vi "VISA MEMACC Read U8 vs U64.vi"() -> ()   [LabVIEW 2016]
uses:
  <vilib>/Platform/TimedLoop/XDataNode/timing_clust.ctl
  <vilib>/Platform/TimedLoop/XDataNode/nitl_modes.ctl
  <vilib>/Platform/TimedLoop/XDataNode/wakeup.ctl
  Source/GE 5565PIORC/GE 5565PIORC Old.lvclass/GE 5565PIORC Old.ctl
  Source/GE 5565PIORC/VIs/Block Operations/Allocate Single Block.vi
  Source/GE 5565PIORC/VIs/Registers/Local Configuration.LAS1RR.Address Range.Get.vi
  Source/GE 5565PIORC/VIs/Binary Operations/Align to 8-byte Boundary.vi
  Source/GE 5565PIORC/VIs/Binary Operations/Align to 16-byte Boundary.vi
  Source/GE 5565PIORC/VIs/Registers/Local Configuration.Get Register Offset.vi
  Source/GE 5565PIORC/GE 5565PIORC Old.lvclass
  <vilib>/platform/TimedLoop/XDataNode/XDataNode.xnode
  <vilib>/Platform/TimedLoop/XDataNode/XDNodeRunTimeDep.lvlib
panel:
  out "U64 Duration":dbl
  in  "U64s":i32
  out "U8 Duration":dbl
  in  "VISA resource name":refnum<visa-resource-name>
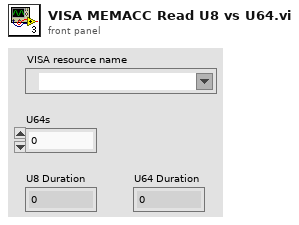
[diagram p1: front panel]
types:
  T1 = typedef "XDNodeRunTimeDep.lvlib/timing_clust.ctl" = cluster{"Expected End [f-1]":u64, "Actual End [f-1]":u64, "Finished Late? [f-1]":bool, "Expected End [i-1]":u64, "Actual End [i-1]":u64, "Finished Late? [i-1]":bool, "Expected Start [i]":u64, "Actual Start [i]":u64, "Expected Start [f]":u64, "Actual Start [f]":u64, "Source Name":string, "Structure Name":string, "Period":i64, "Deadline":i64, "Offset":i64, "Start":i64, "Priority":i32, "Timeout":i32, "Mode":T2, "Wakeup Reason":T3, "Error":errorcluster, "Source Type":string, "Secondary Source Type":string, "Global End Time":u64, "Global Start Time":u64, "Frame Duration":u64, "Iteration Duration":u64, "Assigned CPU":i32, "I/O Scan Engine Mode":u32}
  T2 = typedef "XDNodeRunTimeDep.lvlib/nitl_modes.ctl" = enum32{"No Change", "Process missed periods, maintain original phase", "Discard missed periods, maintain original phase", "Process missed periods, ignore original phase", "Discard missed periods, ignore original phase"}
  T3 = typedef "XDNodeRunTimeDep.lvlib/wakeup.ctl" = enum32{"Normal", "Aborted", "Asynchronous wakeup", "Timing source error", "Timed loop error", "Timeout"}
  T4 = typedef "GE 5565PIORC Old.lvclass/DMA Block Descriptor.ctl" = cluster{"descriptor ptr (VISA)":u32, "descriptor size":u32, "descriptor ptr (aligned)":u32, "data ptr (lower)":u32, "data ptr (upper)":u32, "data size":u32, "next descriptor ptr":u32}
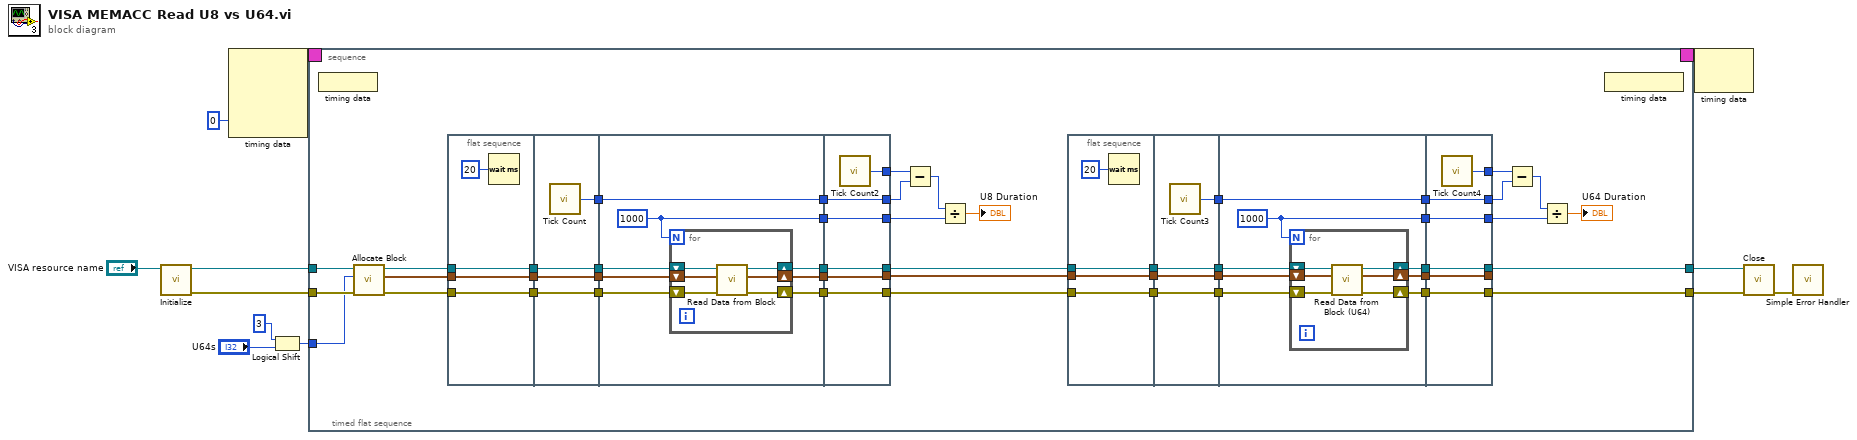
[diagram p0: block diagram]
diagram:
  n1 = call "Initialize.vi"("VISA resource name"="VISA resource name") -> ("error out"=w6:errorcluster, "GE 5565PIORC"=w7:refnum<class "GE 5565PIORC Old.lvclass">)  [unwired: 9 in]
  n2 = node-c288(0 ("Processor")) -> (w10:T1)  [unwired: 3 in]
  n3 = Logical Shift(y=i16 3, x="U64s") -> (x << y=w4:i32)
  n4 = timed-sequence {
    timing: w10 -> [_]
    timing-out: [_] -> w9
    tunnel: w7 -> [w14]
    tunnel: w6 -> [w17]
    tunnel: [w16] -> w1
    tunnel: w4 -> [w15]
    tunnel: [w13] -> w2
    n5 = timed-flat-sequence {
      tunnel: w17 -> [w35]
      tunnel: [w37] -> w16
      tunnel: w15 -> [w32]
      tunnel: w14 -> [w36]
      tunnel: [w18] -> w13
      n6 = node-c288() -> ()  [unwired: 1 in]
      n7 = call-poly "Allocate Block.vi"("error in (no error)"=w35, "size (bytes)"=w32, "GE 5565PIORC in"=w36) -> ("error out"=w33:errorcluster, "Block Descriptor"=w27:T4, "GE 5565PIORC out"=w34:refnum<class "GE 5565PIORC Old.lvclass">)  [unwired: 6 in]
      n8 = flat-sequence {
        tunnel: w34 -> [w93]
        tunnel: w33 -> [w92]
        tunnel: [w93] -> w57
        tunnel: [w92] -> w55
        tunnel: w27 -> [w91]
        tunnel: [w91] -> w26
        tunnel: [w98] -> w62
        tunnel: [w97] -> w58
        tunnel: w57 -> [w97]
        tunnel: [w96] -> w56
        tunnel: w55 -> [w96]
        tunnel: w26 -> [w95]
        tunnel: [w95] -> w25
        tunnel: w62 -> [w106]
        tunnel: [w106] -> w61
        tunnel: w58 -> [w103]
        tunnel: w56 -> [w102]
        tunnel: [w105] -> w54
        tunnel: [w104] -> w53
        tunnel: [w101] -> w31
        tunnel: w25 -> [w100]
        tunnel: [w99] -> w24
        tunnel: [w118] -> w60
        tunnel: [w117] -> w59
        tunnel: w61 -> [w117]
        tunnel: w54 -> [w116]
        tunnel: [w116] -> w38
        tunnel: w53 -> [w115]
        tunnel: [w115] -> w51
        tunnel: w31 -> [w114]
        tunnel: [w114] -> w28
        tunnel: w24 -> [w113]
        tunnel: [w113] -> w23
        frame #0 {
          n9 = Wait (ms)(milliseconds to wait=u32 20) -> ()  [unwired: 1 out]
        }
        frame #1 {
          n10 = call "Tick Count"() -> ("Tick Count(uSec)"=w98:u32)
        }
        frame #2 {
          w104 = 1000
          n11 = for {
            N: w104 -> [_]
            shift-right: [w111] -> w101
            shift-left: w103 -> [w112]
            shift-right: [w109] -> w105
            shift-left: w102 -> [w110]
            shift-right: [w107] -> w99
            shift-left: w100 -> [w108]
            n12 = call "Read Data from Block.vi"("error in (no error)"=w110, "Block Descriptor"=w108, "GE 5565PIORC"=w112) -> ("error out"=w109:errorcluster, "Block Descriptor out"=w107:T4, "GE 5565PIORC out"=w111:refnum<class "GE 5565PIORC Old.lvclass">)  [unwired: 5 in, 1 out]
          }
        }
        frame #3 {
          n13 = call "Tick Count2"() -> ("Tick Count(uSec)"=w118:u32)
        }
      }
      n14 = Subtract(x=w60, y=w59) -> (x-y=w52:u32)
      n15 = Divide(x=w52, y=w51) -> (x/y=→"U8 Duration":dbl)
      n16 = flat-sequence {
        tunnel: w38 -> [w65]
        tunnel: [w65] -> w49
        tunnel: [w64] -> w29
        tunnel: w28 -> [w64]
        tunnel: w23 -> [w63]
        tunnel: [w63] -> w22
        tunnel: [w70] -> w48
        tunnel: [w69] -> w47
        tunnel: w49 -> [w69]
        tunnel: [w68] -> w30
        tunnel: w29 -> [w68]
        tunnel: w22 -> [w67]
        tunnel: [w67] -> w21
        tunnel: w48 -> [w78]
        tunnel: [w78] -> w46
        tunnel: w47 -> [w73]
        tunnel: [w77] -> w45
        tunnel: [w76] -> w44
        tunnel: w30 -> [w75]
        tunnel: w21 -> [w74]
        tunnel: [w72] -> w20
        tunnel: [w71] -> w19
        tunnel: [w90] -> w43
        tunnel: [w89] -> w42
        tunnel: w46 -> [w89]
        tunnel: w45 -> [w88]
        tunnel: [w88] -> w37
        tunnel: w44 -> [w87]
        tunnel: [w87] -> w40
        tunnel: w20 -> [w85]
        tunnel: w19 -> [w86]
        tunnel: [w86] -> w18
        tunnel: [w85] -> _
        frame #0 {
          n17 = Wait (ms)(milliseconds to wait=u32 20) -> ()  [unwired: 1 out]
        }
        frame #1 {
          n18 = call "Tick Count3"() -> ("Tick Count(uSec)"=w70:u32)
        }
        frame #2 {
          w76 = 1000
          n19 = for {
            N: w76 -> [_]
            shift-right: [w81] -> w77
            shift-left: w73 -> [w82]
            shift-right: [w80] -> w71
            shift-left: w75 -> [w84]
            shift-right: [w79] -> w72
            shift-left: w74 -> [w83]
            n20 = call "Read Data from Block (U64).vi"("error in (no error)"=w82, "Block Descriptor"=w83, "GE 5565PIORC"=w84) -> ("error out"=w81:errorcluster, "Block Descriptor out"=w79:T4, "GE 5565PIORC out"=w80:refnum<class "GE 5565PIORC Old.lvclass">)  [unwired: 5 in, 1 out]
          }
        }
        frame #3 {
          n21 = call "Tick Count4"() -> ("Tick Count(uSec)"=w90:u32)
        }
      }
      n22 = Subtract(x=w43, y=w42) -> (x-y=w41:u32)
      n23 = Divide(x=w41, y=w40) -> (x/y=→"U64 Duration":dbl)
      n24 = node-c288() -> ()  [unwired: 1 out]
    }
  }
  n25 = node-c288(w9) -> ()  [unwired: 1 out]
  n26 = call "Close.vi"("error in (no error)"=w1, "GE 5565PIORC in"=w2) -> ("error out"=w11:errorcluster)  [unwired: 8 in, 1 out]
  n27 = call <vilib>:"Simple Error Handler.vi"("error in (no error)"=w11) -> ()  [unwired: 4 in, 5 out]
